vi "ReferencedVariables_AddReferenceVariable.vi"(7 "Action":T2=enum."GeneratePattern", 8 "error in (no error)":errorcluster, 10 "DataIn":variant, 11 "ClassRefToActOn":refnum<vi>) -> (0 "error out":errorcluster, 1 "Name":string, 2 "DataOut":variant, 3 "Cancelled":bool)   [LabVIEW 2014]
uses:
  <resource>/Framework/Providers/Open_GDS/ClassProviders/Provider_BaseClassInterface/BaseProvider_SubVIs/BaseProvider_DesignPatternsActions.ctl
  <resource>/Framework/Providers/Open_GDS/ClassProviders/Common/CommonVIs/CommonVIs_AttributeDataType.ctl
  <resource>/Framework/Providers/Open_GDS/ClassProviders/Common/LvClass_class/GDSLvClass_ProviderTypes.ctl
  <resource>/Framework/Providers/Open_GDS/ClassProviders/Provider_EndevoGOOP300/EndevoProviderName.ctl
  <resource>/Framework/Providers/Open_GDS/ClassProviders/Provider_EndevoGOOP400/EndevoG4ProviderName.ctl
  <resource>/Framework/Providers/Open_GDS/ClassProviders/Provider_LvNativeClass/LvNativeProviderName.ctl
  <resource>/Framework/Providers/Open_GDS/ClassProviders/Common/ScriptingFunctions/Scripting_ConnectorPanePatternType.ctl
  <vilib>/picture/picture.llb/imagedata.ctl
panel:
  in  "_OK+Open":bool
  in  "Delete VI name":string
  in  "Create VI name":string
  out "AlreadyExistsText:VariableName":string
  in  "PlaceInObjectAttribute":bool
  in  "AddViToDelete":bool
  in  "AddViToCreate":bool
  in  "DataType":T1
  in  "Array?":u16(ring) items=["No", "1D", "2D", "3D"]
  in  "Name":string
  in  "_Cancel":bool
  in  "_OK":bool
  out "AlreadyExistsText:Delete":string
  out "AlreadyExistsText:Create":string
  # "Referenced Variables"
  # "Create the variable"
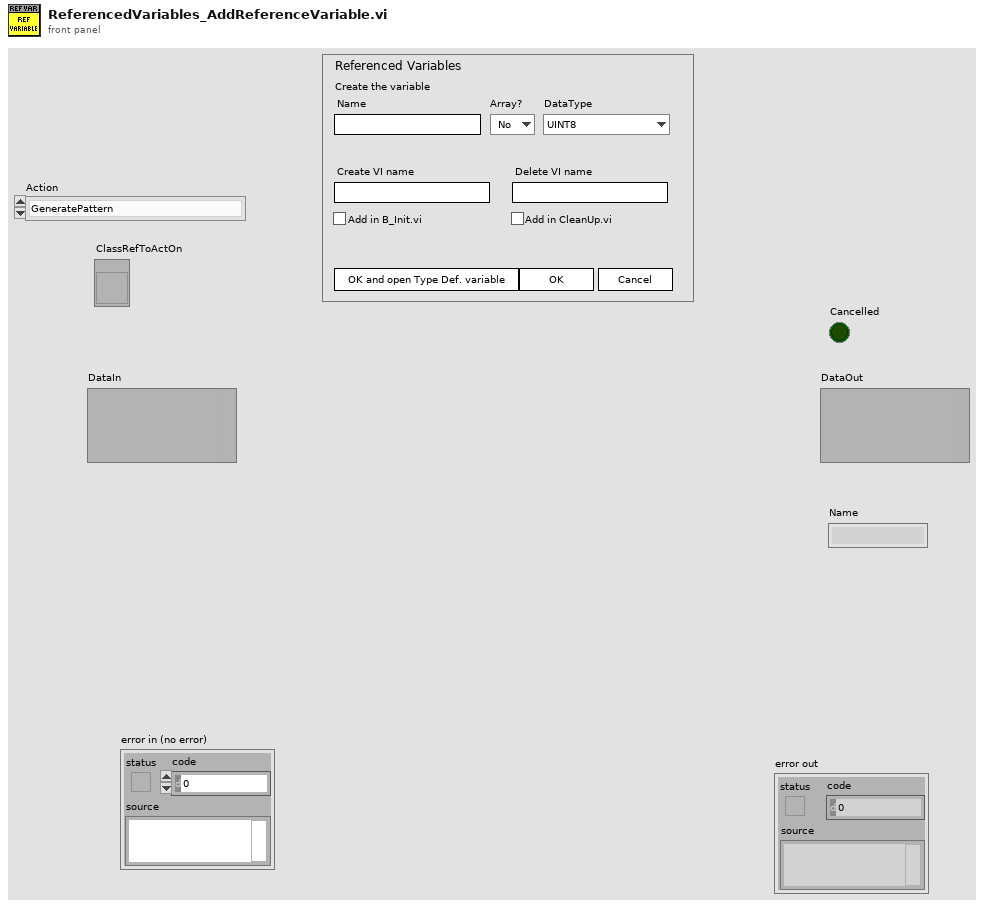
[diagram p1: front panel]
types:
  T1 = typedef "CommonVIs_AttributeDataType.ctl" = enum16{"UINT8", "INT8", "UINT16", "INT16", "UINT32", "INT32", "UINT64", "INT64", "SGL", "DBL", "EXT", "CSG", "CDB", "CXT", "TimeStamp", "STRING", "PATH", "BOOL", "ENUM", "RefNum", "VIRefNum", "LabVIEW Class", "Cluster", "Variant", "TypeDef", "Waveform", "LabVIEW Object", "Other", "void"}
  T2 = typedef "BaseProvider_DesignPatternsActions.ctl" = enum16{"AddPatternDialog", "GeneratePattern", "RemovePattern", "CreatePatternMethod", "UpdatePattern"}
  T3 = cluster{"Name":string, "Array?":u16, "DataType":T1, "Open?":bool, "VarCreateVI":string, "VarDestroyVI":string, "AddViToCreate":bool, "AddViToDelete":bool, "PlaceInObjectAttribute":bool, "ClassCreateVI":string, "ClassDestroyVI":string}
  T4 = typedef "GDSLvClass_ProviderTypes.ctl" = enum16{"UnKnown(LabVOOP)", "Native", "EndevoGOOP3", "OpenG(RootObject)", "OpenG(OpenG_Object)", "EndevoGOOP4", "JKI1"}
  T5 = cluster{"Data":cluster{"Name":string, "Array?":u16, "DataType":T1, "Open?":bool, "VarCreateVI":string, "VarDestroyVI":string, "AddViToCreate":bool, "AddViToDelete":bool, "PlaceInObjectAttribute":bool, "ClassCreateVI":string, "ClassDestroyVI":string}, "SupportFolder":path, "ClassProvider":T4, "ClassName":string, "TemplateName":string, "RefVariablesFolder":path, "Variable.ctl":path, "CreateRefVar.vi":path, "DeleteRefVar.vi":path, "VariablePath":path, "VariableRef":refnum<vi>, "CreateRef":refnum<vi>, "DeleteRef":refnum<vi>, "Application":refnum<vi>, "RefVariablesFolderRef":refnum<vi>, "ClassRef":refnum<vi>, "Singleton":bool, "MethodTemplate":path, "VI":refnum<vi>, "GetObjectStatus":path, "TemplateVI":path, "VI_ToFind":path, "Name":string}
  T6 = enum8{"Enabled", "Disabled", "Disabled and Grayed Out"}
  T7 = typedef "LvNativeProviderName.ctl" = enum16{"Endevo LabVIEW Native"}
  T8 = typedef "EndevoG4ProviderName.ctl" = enum16{"EndevoGOOP400"}
  T9 = typedef "EndevoProviderName.ctl" = enum16{"EndevoGOOP300"}
  T10 = cluster{"Cancelled":bool, "Files":string[], "ClassPath":path, "DataOut":variant, "ByRef":bool, "FilePaths":path[], "CreateVI":string, "DeleteVi":string, "Open?":bool, "Name":string}
  T11 = typedef "imagedata.ctl" = cluster{"image type":i32, "image depth":i32, "image":u8[], "mask":u8[], "colors":u32[], "Rectangle":cluster{"left":i16, "top":i16, "right":i16, "bottom":i16}}
  T12 = typedef "GDSLvCLass_ClassSettingsType.ctl" = cluster{"ClassProviderName":string, "ClassTemplateUsed":string, "ClassTemplateVersion":string, "ClassDescription":string, "PlugIns":T13[], "ConnectorPanePattern":string}
  T13 = typedef "GDSLvClass_PlugIn.ctl" = cluster{"Type":T14, "ID":string, "Version":string, "Path":path, "Name":string, "Data":variant}
  T14 = typedef "GDSLvClass_PlugInTypes.ctl" = enum16{"DesignPattern", "MethodTypes"}
  T15 = typedef "Scripting_ConnectorPanePatternType.ctl" = u16
  T16 = typedef "GDSLvClass_IconSettingsType.ctl" = cluster{"Frame":u32, "Frame thickness":u8, "Header Background":u32, "Header Text":u32, "ColorPublic":u32, "ColorProtected":u32, "ColorPrivate":u32, "Body Text":u32, "ClassBodyIcon":string}
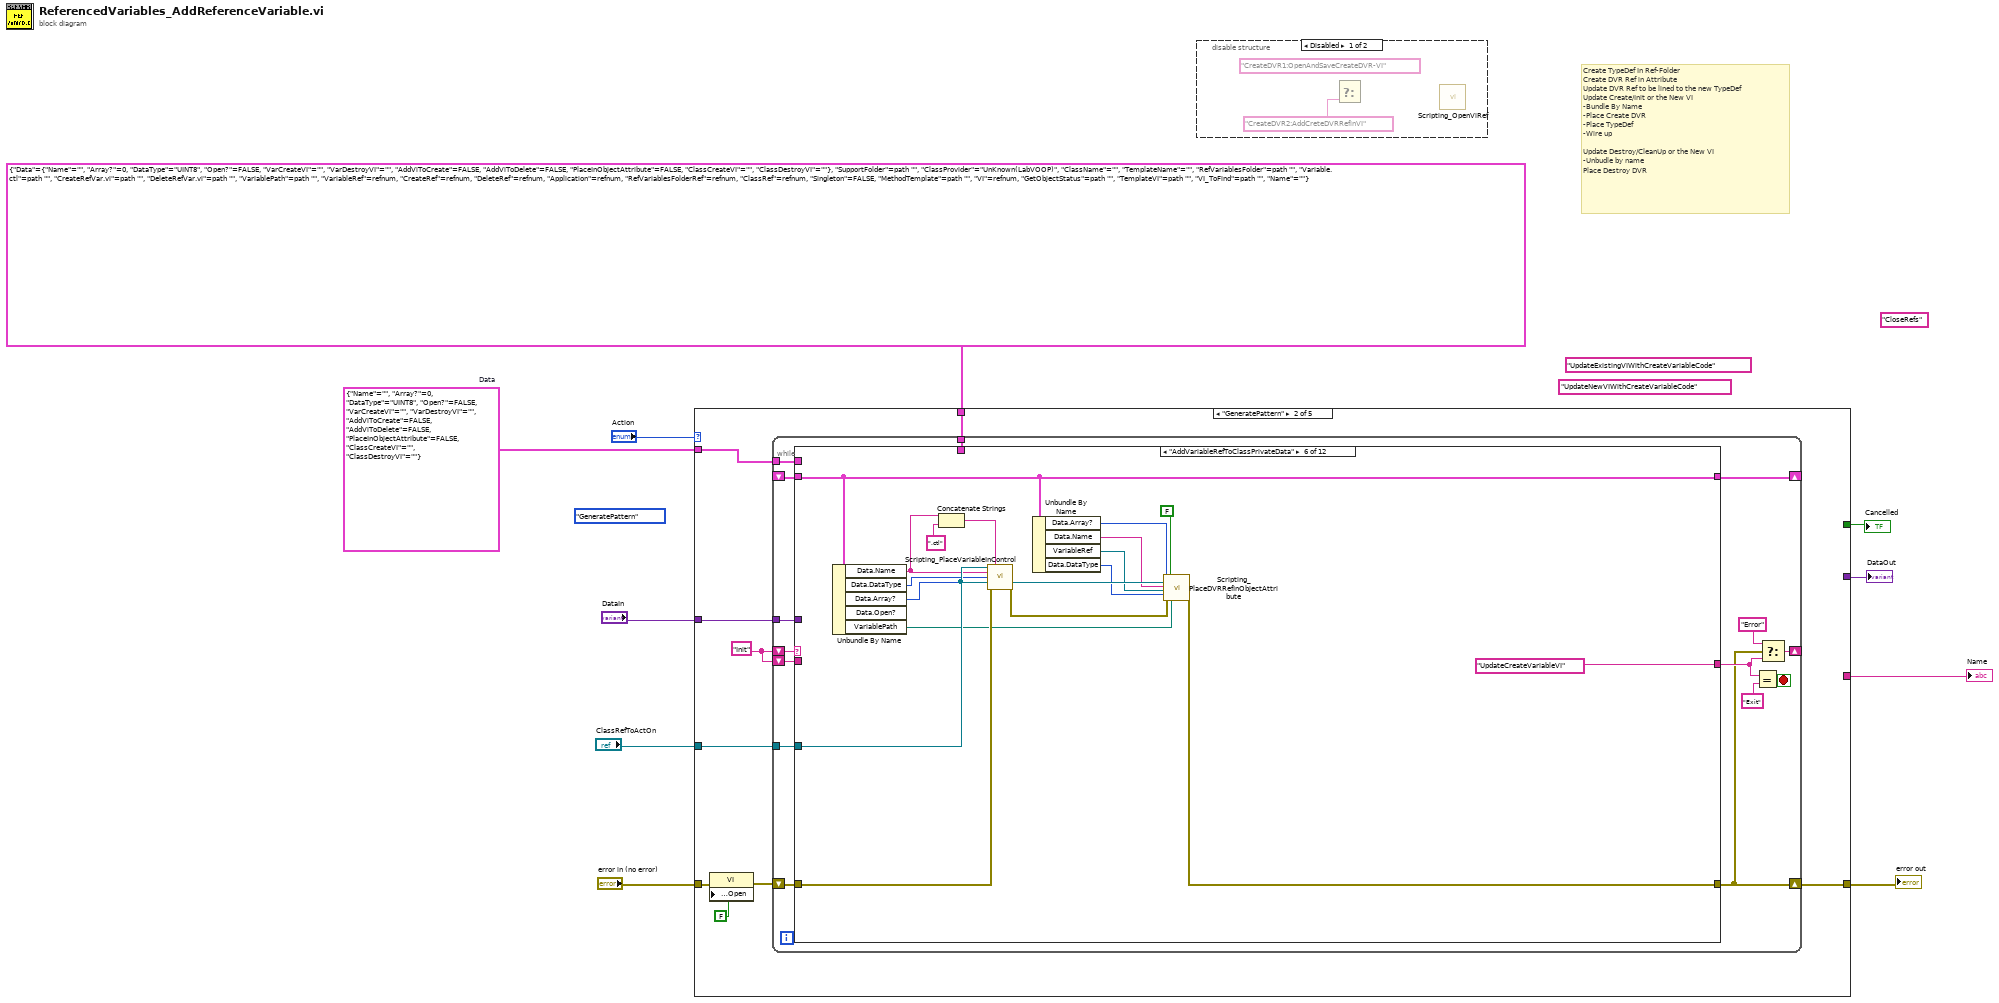
[diagram p0: block diagram]
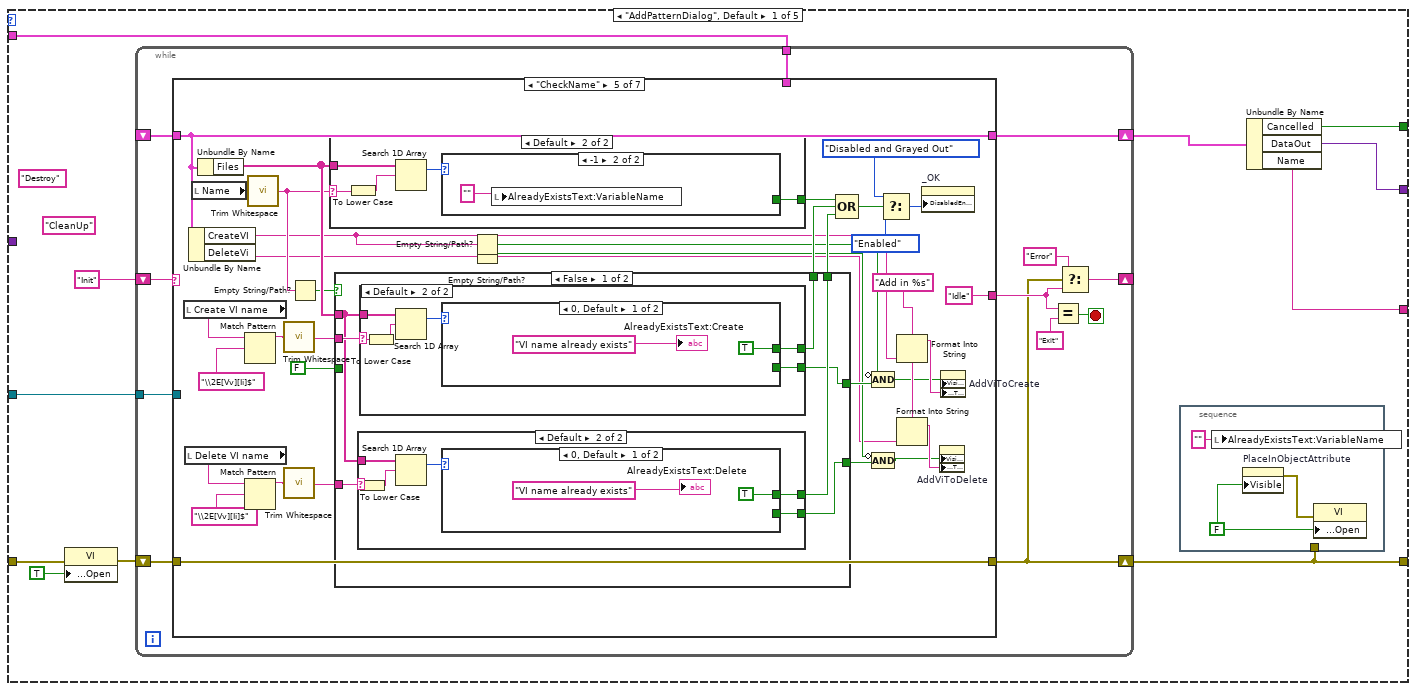
[diagram p3: hidden frame]
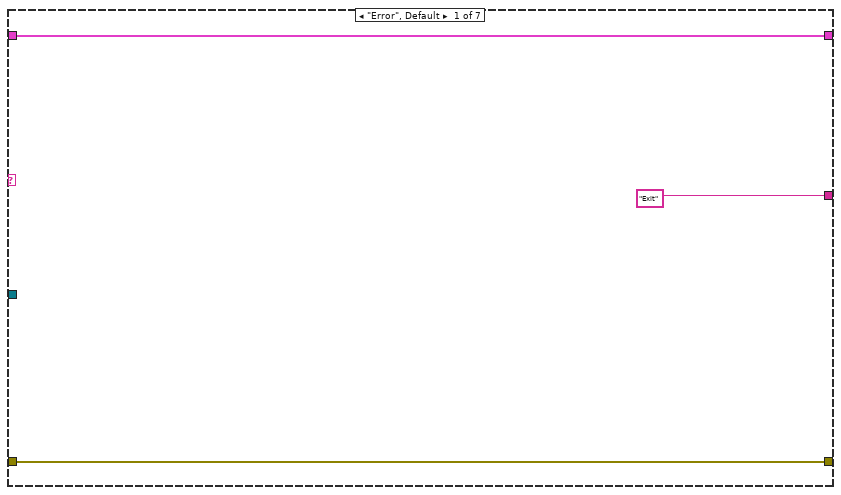
[diagram p4: hidden frame]
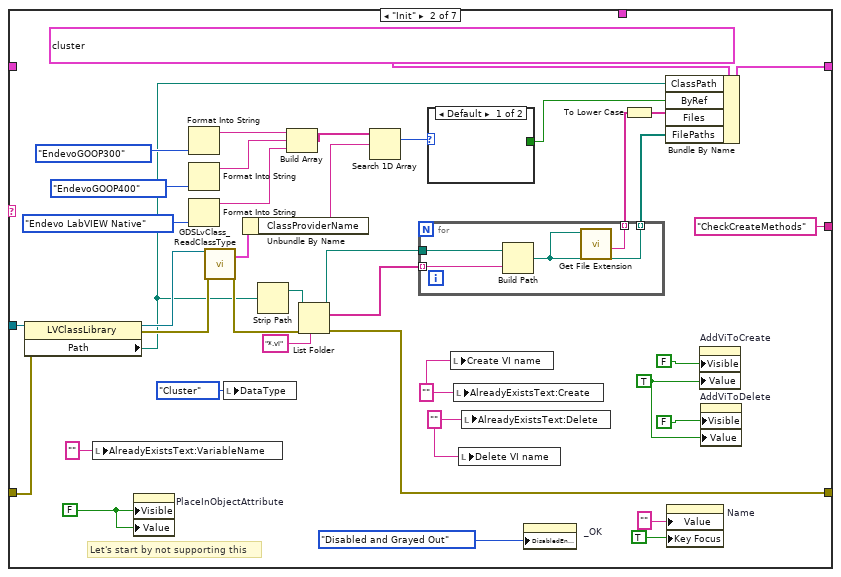
[diagram p5: hidden frame]
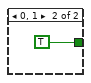
[diagram p6: hidden frame]
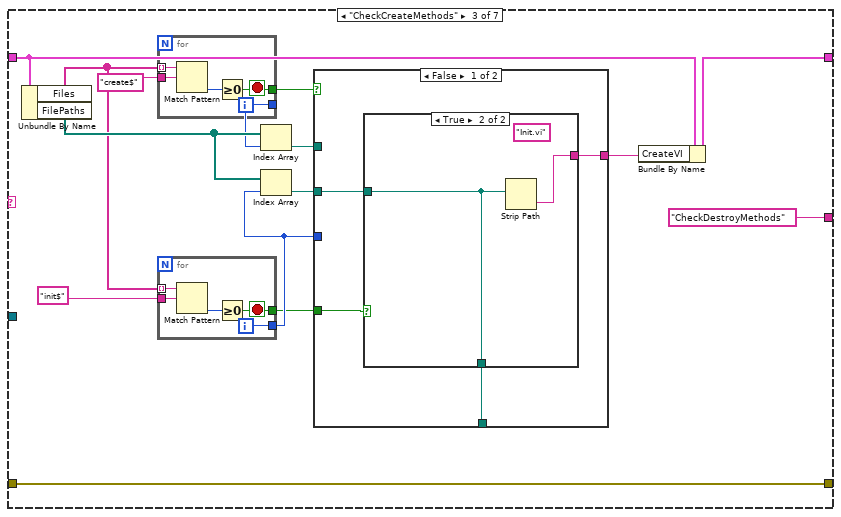
[diagram p7: hidden frame]
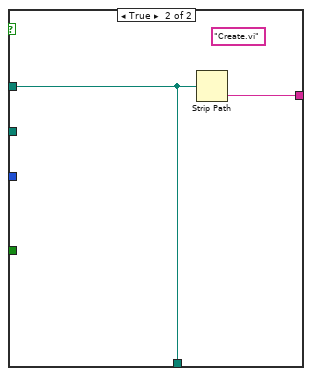
[diagram p9: hidden frame]
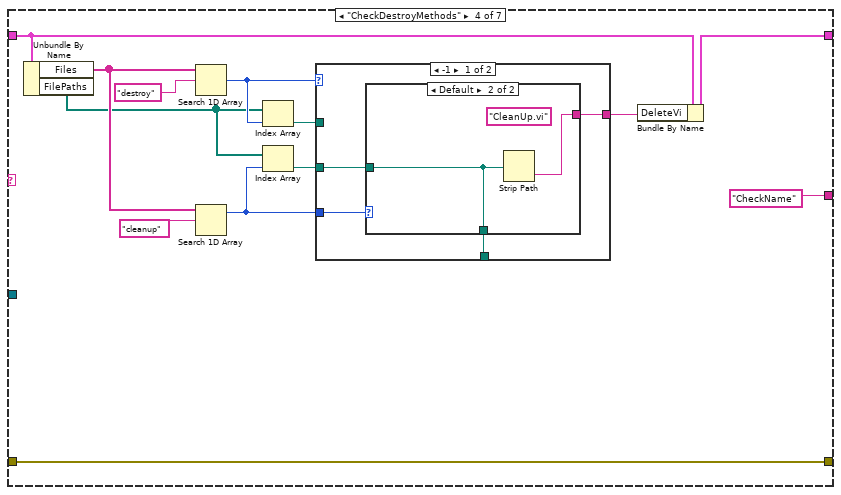
[diagram p10: hidden frame]
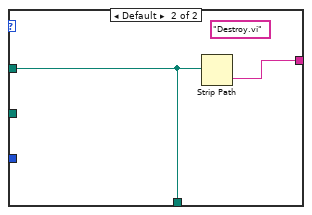
[diagram p12: hidden frame]
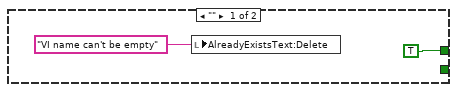
[diagram p13: hidden frame]
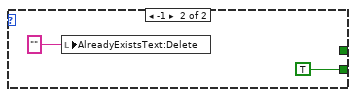
[diagram p14: hidden frame]
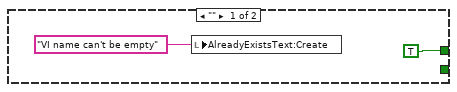
[diagram p15: hidden frame]
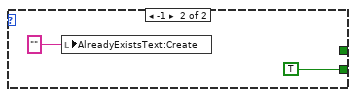
[diagram p16: hidden frame]
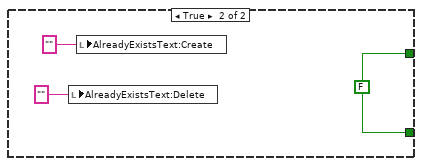
[diagram p17: hidden frame]
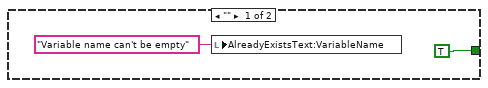
[diagram p18: hidden frame]
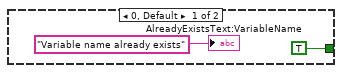
[diagram p19: hidden frame]
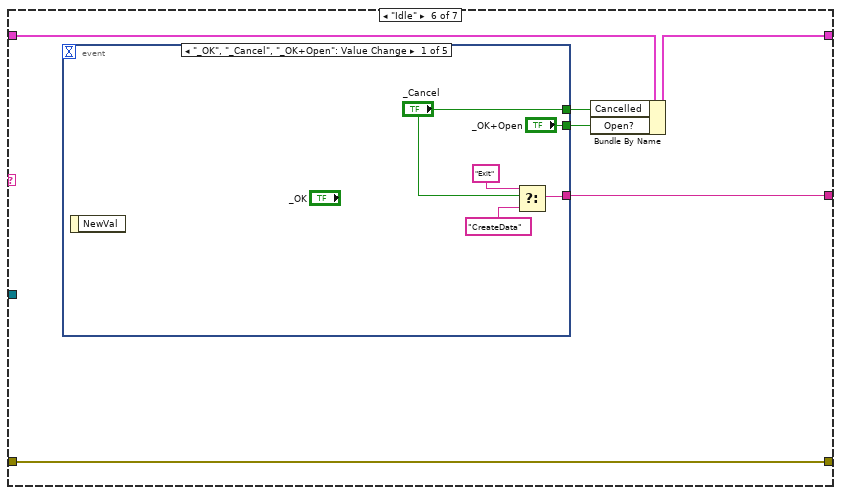
[diagram p20: hidden frame]
diagram:
  (unwired) "CloseRefs"
  (unwired) "UpdateExistingVIWithCreateVariableCode"
  (unwired) "UpdateNewVIWithCreateVariableCode"
  w2 = T3 {"Name"="", "Array?"=0, "DataType"=enum."UINT8", "Open?"=FALSE, "VarCreateVI"="", "VarDestroyVI"="", "AddViToCreate"=FALSE, "AddViToDelete"=FALSE, "PlaceInObjectAttribute"=FALSE, "ClassCreateVI"="", "ClassDestroyVI"=""}  # Data
  (unwired) BaseProvider_DesignPatternsActions."GeneratePattern" ("Action")
  # "Create TypeDef In Ref-Folder\nCreate DVR Ref in Attribute\nUpdate DVR Ref to be lined to the new TypeDef\nUpdate Create/Init or the New VI\n-Bundle By Name\n-Place Create DVR \n-Place TypeDef\n-Wire up\n\nUpdate Destroy/CleanUp or the New VI\n-Unbudle by name\nPlace Destroy DVR"
  n1 = case shown="\"GeneratePattern\"" "Action" {
    tunnel: "error in (no error)" -> [w20 w276 w681 w830 w831]
    tunnel: [w17 w281 w680 w830 w831] -> w9
    tunnel: "ClassRefToActOn" -> [w15 w278 w682 _ _]
    tunnel: [w14 _ _ _ _] -> w7
    tunnel: [w13 _ _ _ _] -> w6
    tunnel: "DataIn" -> [_ w280 w683 _ _]
    tunnel: T5 {"Data"={"Name"="", "Array?"=0, "DataType"=enum."UINT8", "Open?"=FALSE, "VarCreateVI"="", "VarDestroyVI"="", "AddViToCreate"=FALSE, "AddViToDelete"=FALSE, "PlaceInObjectAttribute"=FALSE, "ClassCreateVI"="", "ClassDestroyVI"=""}, "SupportFolder"=path "", "ClassProvider"=enum."UnKnown(LabVOOP)", "ClassName"="", "TemplateName"="", "RefVariablesFolder"=path "", "Variable.ctl"=path "", "CreateRefVar.vi"=path "", "DeleteRefVar.vi"=path "", "VariablePath"=path "", "VariableRef"=refnum, "CreateRef"=refnum, "DeleteRef"=refnum, "Application"=refnum, "RefVariablesFolderRef"=refnum, "ClassRef"=refnum, "Singleton"=FALSE, "MethodTemplate"=path "", "VI"=refnum, "GetObjectStatus"=path "", "TemplateVI"=path "", "VI_ToFind"=path "", "Name"=""} -> [_ w279 w679 _ _]
    tunnel: w2 -> [w12 w273 _ _ _]
    tunnel: [w11 _ _ _ _] -> w1
    frame "AddPatternDialog", Default {
      (unwired) "CleanUp" ("search string")
      (unwired) "Destroy" ("search string")
      n2 = property class="VI"(error in=w20, "Front Panel.Open"=TRUE ("Front Panel Window:Open")) -> (error out=w19:errorcluster)  [unwired: 1 in, 1 out]
      n3 = while {
        shift-right: [w29] -> w17
        shift-left: w19 -> [w36]
        shift-right: [w34] -> _
        shift-left: "Init" -> [w35]
        shift-right: [w28] -> w16
        shift-left: _ -> [w27]
        tunnel: w15 -> [w26]
        tunnel: w12 -> [w25]
        stop <- w33 stop-if-true
        n4 = case shown="\"CheckName\"" w35 {
          tunnel: w36 -> [w39 w74 w90 w118 w171 w220 w270]
          tunnel: [w39 w44 w90 w118 w171 w220 w270] -> w29
          tunnel: ["Exit" "CheckCreateMethods" "CheckDestroyMethods" "CheckName" "Idle" w221 "Exit"] -> w30
          tunnel: [w37 w76 w93 w122 w148 w219 w272] -> w28
          tunnel: w27 -> [w37 _ w94 w123 w148 w217 w245]
          tunnel: w26 -> [_ w75 _ _ _ _ _]
          tunnel: w25 -> [_ _ _ _ _ _ w266]
          frame "Error", Default {
          }
          frame "Init" {
            w50 = "" ("AlreadyExistsText")
            w51 = "" ("AlreadyExistsText")
            w52 = TRUE ("Visible")
            w59 = FALSE ("Visible")
            # "Let's start by not supporting this"
            n5 = property class="LVClassLibrary"(reference=w75, error in=w74) -> (reference out=w72:refnum<vi>, error out=w71:errorcluster, "Path"=w47:path)
            n6 = local write "AlreadyExistsText:VariableName"("" ("AlreadyExistsText")) -> ()
            n7 = property on="PlaceInObjectAttribute" class="Bool (strict)"("Visible"=w59, "Value"=w59) -> ()  [unwired: 2 in, 2 out]
            n8 = Format Into String(EndevoProviderName."EndevoGOOP300" ("ProviderName")) -> (resulting string=w69:string)  [unwired: 3 in, 1 out]
            n9 = Format Into String(EndevoG4ProviderName."EndevoGOOP400" ("ProviderName")) -> (resulting string=w68:string)  [unwired: 3 in, 1 out]
            n10 = Format Into String(LvNativeProviderName."Endevo LabVIEW Native" ("ProviderName")) -> (resulting string=w67:string)  [unwired: 3 in, 1 out]
            n11 = call <resource>:"GDSLvClass_ReadClassType.vi"("Class Refnum In"=w72, "error in (no error)"=w71) -> ("ClassSettings"=w73:T12, "error out"=w49:errorcluster)  [unwired: 15 in, 1 out]
            n12 = local write "DataType"(CommonVIs_AttributeDataType."Cluster" ("DataType")) -> ()
            n13 = Unbundle By Name(w73) -> ("ClassProviderName"=w65:string)
            n14 = Strip Path(path=w47) -> (stripped path=w46:path)  [unwired: 1 out]
            n15 = Build Array(w69, w68, w67) -> (w66:string[])
            n16 = List Folder(path=w46, pattern="*.vi", error in=w49) -> (path out=w45:path, filenames=w42:string[], error out=w44:errorcluster)  [unwired: 1 in, 1 out]
            n17 = Search 1D Array(1D array=w66, element=w65) -> (index of element=w64:i32)  [unwired: 1 in]
            n18 = for {
              tunnel: [w81] -> w58 mode=indexing
              tunnel: w45 -> [w83]
              tunnel: w42 -> [w82] mode=indexing
              tunnel: [w80] -> w41 mode=indexing
              n19 = Build Path(base path=w83, name or relative path=w82) -> (appended path=w81:path)
              n20 = call <vilib>:"Get File Extension.vi"("file"=w81) -> ("filename without extension"=w80:string)  [unwired: 7 in, 3 out]
            }
            n21 = case shown="Default" w64 {
              tunnel: [_ TRUE] -> w61
              frame Default {
              }
              frame 0, 1 {
              }
            }
            n22 = local write "Create VI name"(w51) -> ()
            n23 = local write "AlreadyExistsText:Create"(w51) -> ()
            n24 = local write "Delete VI name"(w50) -> ()
            n25 = local write "AlreadyExistsText:Delete"(w50) -> ()
            n26 = property on="_OK" class="Bool"("DisabledEnum"=T6."Disabled and Grayed Out" ("Disabled")) -> ()  [unwired: 2 in, 2 out]
            n27 = To Lower Case(string=w41) -> (all lower case string=w43:string[])
            n28 = Bundle By Name(cluster=T10 {"Cancelled"=FALSE, "Files"=[], "ClassPath"=path "", "DataOut"=variant, "ByRef"=FALSE, "FilePaths"=[], "CreateVI"="", "DeleteVi"="", "Open?"=TRUE, "Name"=""}, "ClassPath"=w47, "ByRef"=w61, "Files"=w43, "FilePaths"=w58) -> (w76:T10)
            n29 = property on="Name" class="Str"("Value"="" ("AlreadyExistsText"), "Key Focus"=TRUE) -> ()  [unwired: 2 in, 2 out]
            n30 = property on="AddViToCreate" class="Bool (strict)"("Visible"=FALSE, "Value"=w52) -> ()  [unwired: 2 in, 2 out]
            n31 = property on="AddViToDelete" class="Bool (strict)"("Visible"=FALSE, "Value"=w52) -> ()  [unwired: 2 in, 2 out]
          }
          frame "CheckCreateMethods" {
            n32 = Unbundle By Name(w94) -> ("Files"=w87:string[], "FilePaths"=w96:path[])
            n33 = for {
              tunnel: w87 -> [w108] mode=indexing
              tunnel: "create$" ("search string") -> [w107]
              tunnel: [w105] -> w91
              tunnel: [w104] -> w88
              i -> [w105]
              stop <- w104 stop-if-true
              n34 = Match Pattern(string=w108, regular expression=w107) -> (offset past match=w106:i32)  [unwired: 1 in, 3 out]
              n35 = Greater Or Equal To 0?(x=w106) -> (x >= 0?=w104:bool)
            }
            n36 = for {
              tunnel: w87 -> [w103] mode=indexing
              tunnel: "init$" ("search string") -> [w102]
              tunnel: [w100] -> w85
              tunnel: [w99] -> w84
              i -> [w100]
              stop <- w99 stop-if-true
              n37 = Match Pattern(string=w103, regular expression=w102) -> (offset past match=w101:i32)  [unwired: 1 in, 3 out]
              n38 = Greater Or Equal To 0?(x=w101) -> (x >= 0?=w99:bool)
            }
            n39 = Index Array(array=w96, index=w91) -> (element=w97:path)
            n40 = Index Array(array=w96, index=w85) -> (element=w95:path)
            n41 = case shown="False" w88 {
              tunnel: w85 -> [_ _]
              tunnel: [w111 w116] -> _
              tunnel: w97 -> [_ w116]
              tunnel: w95 -> [w112 _]
              tunnel: [w110 w115] -> w89
              tunnel: w84 -> [w109 _]
              frame False {
                n42 = case shown="True" w109 {
                  tunnel: w112 -> [_ w114]
                  tunnel: [_ w114] -> w111
                  tunnel: [_ w113] -> w110
                  frame False {
                  }
                  frame True {
                    (unwired) "Init.vi" ("search string")
                    n43 = Strip Path(path=w114) -> (name=w113:string)  [unwired: 1 out]
                  }
                }
              }
              frame True {
                (unwired) "Create.vi" ("search string")
                n44 = Strip Path(path=w116) -> (name=w115:string)  [unwired: 1 out]
              }
            }
            n45 = Bundle By Name(cluster=w94, "CreateVI"=w89) -> (w93:T10)
          }
          frame "CheckDestroyMethods" {
            n46 = Unbundle By Name(w123) -> ("Files"=w128:string[], "FilePaths"=w120:path[])
            n47 = Search 1D Array(1D array=w128, element="destroy" ("search string")) -> (index of element=w125:i32)  [unwired: 1 in]
            n48 = Search 1D Array(1D array=w128, element="cleanup" ("search string")) -> (index of element=w121:i32)  [unwired: 1 in]
            n49 = Index Array(array=w120, index=w125) -> (element=w124:path)
            n50 = Index Array(array=w120, index=w121) -> (element=w119:path)
            n51 = case shown="-1" w125 {
              tunnel: w121 -> [w133 _]
              tunnel: [w131 w137] -> _
              tunnel: w124 -> [_ w137]
              tunnel: w119 -> [w132 _]
              tunnel: [w130 w136] -> w117
              frame -1 {
                n52 = case shown="Default" w133 {
                  tunnel: w132 -> [_ w135]
                  tunnel: [_ w135] -> w131
                  tunnel: [_ w134] -> w130
                  frame -1 {
                  }
                  frame Default {
                    (unwired) "CleanUp.vi" ("search string")
                    n53 = Strip Path(path=w135) -> (name=w134:string)  [unwired: 1 out]
                  }
                }
              }
              frame Default {
                (unwired) "Destroy.vi" ("search string")
                n54 = Strip Path(path=w137) -> (name=w136:string)  [unwired: 1 out]
              }
            }
            n55 = Bundle By Name(cluster=w123, "DeleteVi"=w117) -> (w122:T10)
          }
          frame "CheckName" {
            w151 = "Add in %s" ("format string")
            n56 = local read "Create VI name"() -> (w141:string)
            n57 = local read "Delete VI name"() -> (w138:string)
            n58 = Unbundle By Name(w148) -> ("CreateVI"=w140:string, "DeleteVi"=w139:string)
            n59 = local read "Name"() -> (w162:string)
            n60 = Unbundle By Name(w148) -> ("Files"=w155:string[])
            n61 = Match Pattern(string=w141, regular expression="\\2E[Vv][Ii]$") -> (before substring=w163:string)  [unwired: 1 in, 3 out]
            n62 = Match Pattern(string=w138, regular expression="\\2E[Vv][Ii]$") -> (before substring=w159:string)  [unwired: 1 in, 3 out]
            n63 = call <vilib>:"Trim Whitespace.vi"("string"=w162) -> ("trimmed string"=w154:string)  [unwired: 1 in]
            n64 = call <vilib>:"Trim Whitespace.vi"("string"=w163) -> ("trimmed string"=w161:string)  [unwired: 1 in]
            n65 = call <vilib>:"Trim Whitespace.vi"("string"=w159) -> ("trimmed string"=w160:string)  [unwired: 1 in]
            n66 = Empty String/Path?(string/path=w154) -> (empty?=w153:bool)
            n67 = case shown="Default" w154 {
              selector: w154 -> [_ w208]
              tunnel: w155 -> [_ w210]
              tunnel: [TRUE w209] -> w168
              frame "" {
                n68 = local write "AlreadyExistsText:VariableName"("Variable name can't be empty" ("AlreadyExistsText")) -> ()
              }
              frame Default {
                n69 = To Lower Case(string=w208) -> (all lower case string=w211:string)
                n70 = Search 1D Array(1D array=w210, element=w211) -> (index of element=w212:i32)  [unwired: 1 in]
                n71 = case shown="-1" w212 {
                  tunnel: [TRUE _] -> w209
                  frame 0, Default {
                    "AlreadyExistsText:VariableName" <- "Variable name already exists" ("AlreadyExistsText")
                  }
                  frame -1 {
                    n72 = local write "AlreadyExistsText:VariableName"("" ("AlreadyExistsText")) -> ()
                  }
                }
              }
            }
            n73 = case shown="False" w153 {
              tunnel: w161 -> [w178 _]
              tunnel: w160 -> [w177 _]
              tunnel: [w176 _] -> w157
              tunnel: [w175 _] -> w156
              tunnel: w155 -> [w174 _]
              tunnel: FALSE ("x = 0?") -> [_ _]
              tunnel: [w173 w203] -> w147
              tunnel: [w172 w203] -> w144
              frame False {
                n74 = case shown="Default" w177 {
                  selector: w177 -> [_ w182]
                  tunnel: w174 -> [_ w184]
                  tunnel: [TRUE w183] -> w175
                  tunnel: [_ w181] -> w172
                  frame "" {
                    n75 = local write "AlreadyExistsText:Delete"("VI name can't be empty" ("AlreadyExistsText")) -> ()
                  }
                  frame Default {
                    n76 = To Lower Case(string=w182) -> (all lower case string=w185:string)
                    n77 = Search 1D Array(1D array=w184, element=w185) -> (index of element=w186:i32)  [unwired: 1 in]
                    n78 = case shown="0, Default" w186 {
                      tunnel: [TRUE _] -> w183
                      tunnel: [_ TRUE] -> w181
                      frame 0, Default {
                        "AlreadyExistsText:Delete" <- "VI name already exists" ("AlreadyExistsText")
                      }
                      frame -1 {
                        n79 = local write "AlreadyExistsText:Delete"("" ("AlreadyExistsText")) -> ()
                      }
                    }
                  }
                }
                n80 = case shown="Default" w178 {
                  selector: w178 -> [_ w194]
                  tunnel: w174 -> [_ w196]
                  tunnel: [TRUE w195] -> w176
                  tunnel: [_ w193] -> w173
                  frame "" {
                    n81 = local write "AlreadyExistsText:Create"("VI name can't be empty" ("AlreadyExistsText")) -> ()
                  }
                  frame Default {
                    n82 = To Lower Case(string=w194) -> (all lower case string=w197:string)
                    n83 = Search 1D Array(1D array=w196, element=w197) -> (index of element=w198:i32)  [unwired: 1 in]
                    n84 = case shown="0, Default" w198 {
                      tunnel: [TRUE _] -> w195
                      tunnel: [_ TRUE] -> w193
                      frame 0, Default {
                        "AlreadyExistsText:Create" <- "VI name already exists" ("AlreadyExistsText")
                      }
                      frame -1 {
                        n85 = local write "AlreadyExistsText:Create"("" ("AlreadyExistsText")) -> ()
                      }
                    }
                  }
                }
              }
              frame True {
                w203 = FALSE
                n86 = local write "AlreadyExistsText:Delete"("" ("AlreadyExistsText")) -> ()
                n87 = local write "AlreadyExistsText:Create"("" ("AlreadyExistsText")) -> ()
              }
            }
            n88 = Empty String/Path?(string/path=w140) -> (empty?=w145:bool)
            n89 = Empty String/Path?(string/path=w139) -> (empty?=w142:bool)
            n90 = Compound Arithmetic op=OR(w168, w157, w156) -> (w167:bool)
            n91 = Compound Arithmetic op=AND(invert w145, w147) -> (w146:bool)
            n92 = Compound Arithmetic op=AND(invert w142, w144) -> (w143:bool)
            n93 = Select(t=T6."Disabled and Grayed Out" ("Disabled"), s=w167, f=T6."Enabled" ("Disabled")) -> (s? t:f=w164:T6)
            n94 = Format Into String(format string=w151, w140) -> (resulting string=w150:string)  [unwired: 2 in, 1 out]
            n95 = Format Into String(format string=w151, w139) -> (resulting string=w149:string)  [unwired: 2 in, 1 out]
            n96 = property on="_OK" class="Bool"("DisabledEnum"=w164) -> ()  [unwired: 2 in, 2 out]
            n97 = property on="AddViToDelete" class="Bool (strict)"("Visible"=w143, "BoolText.Text"=w149) -> ()  [unwired: 2 in, 2 out]
            n98 = property on="AddViToCreate" class="Bool (strict)"("Visible"=w146, "BoolText.Text"=w150) -> ()  [unwired: 2 in, 2 out]
          }
          frame "Idle" {
            n99 = event shown="[0] \"_OK\", \"_Cancel\", \"_OK+Open\": Value Change" {
              selector: _ -> [_ _ _ _ _]
              dyn-events: _ -> [_ _ _ _ _]
              timeout: _ -> [_ _ _ _ _]
              tunnel: [w226 "Exit" "CheckName" "CheckName" "CheckName"] -> w221
              tunnel: ["_Cancel" w227 _ _ _] -> w218
              tunnel: ["_OK+Open" _ _ _ _] -> w216
              event "_OK", "_Cancel", "_OK+Open": Value Change {
                n100 = event-data() -> ()  [unwired: 1 in, 1 out]
                n101 = Select(t="Exit", s="_Cancel", f="CreateData") -> (s? t:f=w226:string)
              }
              event Panel Close? {
                w227 = TRUE ("Discard?")
                n102 = event-data() -> ()  [unwired: 1 in, 1 out]
                n103 = event-data("Discard?"=w227) -> ()  [unwired: 1 in, 1 out]
              }
              event "Name": Value Change {
                n104 = event-data() -> ()  [unwired: 1 in, 1 out]
                n105 = Empty String/Path?(string/path="Name") -> (empty?=w229:bool)
                n106 = case shown="False" w229 {
                  tunnel: [w239 _] -> w232
                  tunnel: [w238 _] -> w231
                  tunnel: "Name" -> [w236 _]
                  frame False {
                    n107 = Concatenate Strings("Create" ("string"), w236, "Ref" ("string")) -> (w239:string)
                    n108 = Concatenate Strings("Delete" ("string"), w236, "Ref" ("string")) -> (w238:string)
                  }
                  frame True {
                  }
                }
                n109 = local write "Delete VI name"(w231) -> ()
                n110 = local write "Create VI name"(w232) -> ()
              }
              event "Create VI name", "Delete VI name": Value Change {
                n111 = event-data() -> ()  [unwired: 1 in, 1 out]
              }
              event "AddViToDelete", "AddViToCreate": Value Change {
                n112 = event-data() -> ()  [unwired: 1 in, 1 out]
              }
            }
            n113 = Bundle By Name(cluster=w217, "Cancelled"=w218, "Open?"=w216) -> (w219:T10)
          }
          frame "CreateData" {
            # "Hidden for now"
            n114 = Unbundle By Name(w245) -> ("Open?"=w244:bool)
            n115 = local read "Create VI name"() -> (w263:string)
            n116 = local read "Delete VI name"() -> (w257:string)
            n117 = local read "AddViToDelete"() -> (w250:bool)
            n118 = Unbundle By Name(w245) -> ("CreateVI"=w247:string, "DeleteVi"=w246:string)
            n119 = local read "AddViToCreate"() -> (w251:bool)
            n120 = local read "Name"() -> (w265:string)
            n121 = call <vilib>:"Trim Whitespace.vi"("string"=w263) -> ("trimmed string"=w262:string)  [unwired: 1 in]
            n122 = call <vilib>:"Trim Whitespace.vi"("string"=w257) -> ("trimmed string"=w256:string)  [unwired: 1 in]
            n123 = Match Pattern(string=w262, regular expression="\\2E[Vv][Ii]$") -> (before substring=w261:string)  [unwired: 1 in, 3 out]
            n124 = Match Pattern(string=w256, regular expression="\\2E[Vv][Ii]$") -> (before substring=w255:string)  [unwired: 1 in, 3 out]
            n125 = call <vilib>:"Trim Whitespace.vi"("string"=w265) -> ("trimmed string"=w243:string)  [unwired: 1 in]
            n126 = call <vilib>:"Trim Whitespace.vi"("string"=w261) -> ("trimmed string"=w260:string)  [unwired: 1 in]
            n127 = call <vilib>:"Trim Whitespace.vi"("string"=w255) -> ("trimmed string"=w254:string)  [unwired: 1 in]
            n128 = Concatenate Strings(w260, ".vi" ("string")) -> (w248:string)
            n129 = Concatenate Strings(w254, ".vi" ("string")) -> (w252:string)
            n130 = Bundle(cluster=w266, "Name"=w243, "Array?"="Array?", "DataType"="DataType", "Open?"=w244, "VarCreateVI"=w248, "VarDestroyVI"=w252, "AddViToCreate"=w251, "AddViToDelete"=w250, "PlaceInObjectAttribute"="PlaceInObjectAttribute", "ClassCreateVI"=w247, "ClassDestroyVI"=w246) -> (w267:T3)
            n131 = Bundle By Name(cluster=w245, "Name"=w243, "DataOut"=w267) -> (w272:T10)
          }
        }
        n132 = Equal?(x=w30, y="Exit") -> (x = y?=w33:bool)
        n133 = Select(t="Error", s=w29, f=w30) -> (s? t:f=w34:string)
      }
      n134 = stacked-sequence {
        tunnel: w17 -> [_]
        frame #0 {
          w24 = FALSE ("Front Panel Window:Open")
          n135 = local write "AlreadyExistsText:VariableName"("" ("AlreadyExistsText")) -> ()
          n136 = property on="PlaceInObjectAttribute" class="Bool (strict)"("Visible"=w24) -> (error out=w23:errorcluster)  [unwired: 2 in, 1 out]
          n137 = property class="VI"(error in=w23, "Front Panel.Open"=w24) -> ()  [unwired: 1 in, 2 out]
        }
      }
      n138 = Unbundle By Name(w16) -> ("Cancelled"=w14:bool, "DataOut"=w13:variant, "Name"=w11:string)
    }
    frame "GeneratePattern" {
      w274 = "Init"
      n139 = property class="VI"(error in=w276, "Front Panel.Open"=FALSE ("Front Panel Window:Open")) -> (error out=w275:errorcluster)  [unwired: 1 in, 1 out]
      n140 = while {
        shift-right: [w289] -> w281
        shift-left: w275 -> [w296]
        shift-right: [w294] -> _
        shift-left: w274 -> [w295]
        shift-right: [w288] -> _
        shift-left: _ -> [w287]
        tunnel: w280 -> [w286]
        tunnel: w273 -> [w285]
        tunnel: w279 -> [w284]
        tunnel: w278 -> [w283]
        shift-left: w274 -> [w282]
        stop <- w293 stop-if-true
        n141 = case shown="\"AddVariableRefToClassPrivateData\"" w295 {
          tunnel: w296 -> [w321 w363 w379 w395 w412 w430 w456 w486 w500 w541 w595 w661]
          tunnel: [w302 w358 w375 w389 w404 w429 w436 w467 w499 w540 w594 w665] -> w289
          tunnel: ["GetTemplateVIs" "OpenTemplateVIs" "SaveVIToNewName" "AddVIsToClass" "AddVariableRefToClassPrivateData" "UpdateCreateVariableVI" "UpdateDeleteVariableVI" "UpdateIcons" "AddCreateVariableVIInCreate" "AddDeleteVariableVIInDestroy" "CloseRefs" "Exit"] -> w290
          tunnel: [w325 w348 w370 w386 w402 w414 w443 w474 w501 w536 w590 w663] -> w288
          tunnel: w287 -> [_ w362 w369 w387 w402 w414 w443 w474 w501 w536 w590 w663]
          tunnel: w286 -> [w324 _ _ _ _ _ _ _ _ _ _ _]
          tunnel: w285 -> [w323 _ _ _ _ _ _ _ _ _ _ _]
          tunnel: w284 -> [w322 _ _ _ _ _ _ _ _ _ _ _]
          tunnel: w283 -> [w320 w364 _ _ _ w428 _ _ w503 w537 w591 w659]
          tunnel: w282 -> [_ _ _ _ _ _ _ _ _ _ _ w662]
          frame "Init" {
            w300 = "ReferencedVariables" ("name or relative path")
            n142 = Variant To Data(error in=w321, type=w323, Variant=w324) -> (data=w306:T3, error out=w315:errorcluster)
            n143 = property class="LVClassLibrary"(reference=w320, error in=w315) -> (reference out=w297:refnum<vi>, error out=w307:errorcluster, "Path"=w314:path)
            n144 = property class="LVClassLibrary"(reference=w297, error in=w307) -> (reference out=w311:refnum<vi>, error out=w309:errorcluster, "Target"=w310:refnum<vi>)
            n145 = Current VI's Path() -> (path=w318:path)
            n146 = Strip Path(path=w318) -> (stripped path=w317:path)  [unwired: 1 out]
            n147 = To More Generic Class(target class=refnum<vi> refnum ("AddItem"), reference=w297) -> (generic class reference=w301:refnum<vi>)
            n148 = Strip Path(path=w314) -> (stripped path=w305:path, name=w312:string)
            n149 = Build Path(base path=w317, name or relative path="ReferencedVariables_SubVIs") -> (appended path=w313:path)
            n150 = case shown="Error" w309 {
              selector: w309 -> [w328 _]
              tunnel: w310 -> [w332 _]
              tunnel: [w331 w334] -> w308
              tunnel: [w327 w335] -> w303
              tunnel: w311 -> [_ w340]
              tunnel: w307 -> [_ w339]
              frame No Error {
                n151 = property class="TargetItem"(reference=w332, error in=w328) -> (reference out=w329:refnum<vi>, error out=w330:errorcluster, "Context"=w331:refnum<vi>)
                n152 = Close Reference(reference=w329, error in (no error)=w330) -> (error out=w327:errorcluster)
              }
              frame Error {
                n153 = property class="LVClassLibrary"(reference=w340, error in=w339) -> (error out=w333:errorcluster, "Project"=w338:refnum<vi>)  [unwired: 1 out]
                n154 = property class="Project"(reference=w338, error in=w333) -> (reference out=w336:refnum<vi>, error out=w337:errorcluster, "App Ref"=w334:refnum<vi>)
                n155 = Close Reference(reference=w336, error in (no error)=w337) -> (error out=w335:errorcluster)
              }
            }
            n156 = Build Path(base path=w305, name or relative path=w300) -> (appended path=w304:path)
            n157 = call <resource>:"GDSProject_CreateFolder.vi"("Project Item To Create Folder Below(Use MyComputer if not wired)"=w301, "FolderName"=w300, "error in (no error)"=w303, "CreateThePhysicalFolderIfPossible(False)"=TRUE) -> ("ItemOut"=w299:refnum<vi>, "error out"=w302:errorcluster)  [unwired: 12 in, 2 out]
            n158 = Bundle By Name(cluster=w322, "Data"=w306, "SupportFolder"=w313, "ClassName"=w312, "RefVariablesFolder"=w304, "RefVariablesFolderRef"=w299, "Application"=w308, "ClassRef"=w297) -> (w325:T5)
          }
          frame "GetTemplateVIs" {
            w354 = T15 0 items=["4x4x4", "5x6x5", "6x8x6"] ("Pattern")
            n159 = call <resource>:"GDSLvClass_GetClassProviderInformation.vi"("Class Refnum In"=w364, "error in (no error)"=w363) -> ("Class Refnum Out"=w360:refnum<vi>, "ClassProvider"=w361:T4, "error out"=w359:errorcluster)  [unwired: 15 in]
            n160 = Unbundle By Name(w362) -> ("SupportFolder"=w344:path)
            n161 = call <resource>:"GDSLvClass_ReadClassType.vi"("Class Refnum In"=w360, "error in (no error)"=w359) -> ("ClassSettings"=w357:T12, "error out"=w358:errorcluster)  [unwired: 15 in, 1 out]
            n162 = Unbundle By Name(w357) -> ("ConnectorPanePattern"=w350:string, "ClassTemplateUsed"=w356:string)
            n163 = Scan From String(input string=w350, default 1=w354) -> (output 1=w351:T15)  [unwired: 3 in, 3 out]
            n164 = case shown="Default" w351 {
              tunnel: ["4x4x4" "6x8x6"] -> w346
              frame 0 {
              }
              frame Default {
              }
            }
            n165 = Format Into String(format string="ReferencedVariables_CreateReferenceVariable_%s.vi" ("name or relative path"), w346) -> (resulting string=w352:string)  [unwired: 2 in, 1 out]
            n166 = Format Into String(format string="ReferencedVariables_DeleteReferenceVariable_%s.vi" ("name or relative path"), w346) -> (resulting string=w343:string)  [unwired: 2 in, 1 out]
            n167 = Build Path(base path=w344, name or relative path="ReferencedVariable.ctl") -> (appended path=w355:path)
            n168 = Build Path(base path=w344, name or relative path=w352) -> (appended path=w345:path)
            n169 = Build Path(base path=w344, name or relative path=w343) -> (appended path=w342:path)
            n170 = Bundle By Name(cluster=w362, "Variable.ctl"=w355, "ClassProvider"=w361, "CreateRefVar.vi"=w345, "DeleteRefVar.vi"=w342, "TemplateName"=w356) -> (w348:T5)
          }
          frame "OpenTemplateVIs" {
            n171 = Unbundle By Name(w369) -> ("Application"=w376:refnum<vi>, "Variable.ctl"=w380:path)
            n172 = Unbundle By Name(w369) -> ("CreateRefVar.vi"=w368:path)
            n173 = Unbundle By Name(w369) -> ("DeleteRefVar.vi"=w367:path)
            n174 = Open VI Reference(application reference (local)=w376, vi path=w380, error in (no error)=w379) -> (vi reference=w373:refnum<vi>, error out=w378:errorcluster)  [unwired: 3 in]
            n175 = Open VI Reference(application reference (local)=w376, vi path=w368, error in (no error)=w378) -> (vi reference=w372:refnum<vi>, error out=w377:errorcluster)  [unwired: 3 in]
            n176 = Open VI Reference(application reference (local)=w376, vi path=w367, error in (no error)=w377) -> (vi reference=w371:refnum<vi>, error out=w375:errorcluster)  [unwired: 3 in]
            n177 = Bundle By Name(cluster=w369, "VariableRef"=w373, "CreateRef"=w372, "DeleteRef"=w371) -> (w370:T5)
          }
          frame "SaveVIToNewName" {
            n178 = Unbundle By Name(w387) -> ("VariableRef"=w399:refnum<vi>, "RefVariablesFolder"=w384:path, "Data.Name"=w398:string)
            n179 = Unbundle By Name(w387) -> ("CreateRef"=w393:refnum<vi>, "Data.VarCreateVI"=w385:string)
            n180 = Unbundle By Name(w387) -> ("DeleteRef"=w392:refnum<vi>, "Data.VarDestroyVI"=w383:string)
            n181 = Concatenate Strings(w398, ".ctl" ("string")) -> (w396:string)
            n182 = Build Path(base path=w384, name or relative path=w396) -> (appended path=w388:path)
            n183 = Build Path(base path=w384, name or relative path=w385) -> (appended path=w382:path)
            n184 = Build Path(base path=w384, name or relative path=w383) -> (appended path=w381:path)
            n185 = invoke class="VI" method="Save.Instrument"(reference=w399, error in=w395, "Path to saved file"=w388) -> (error out=w394:errorcluster)  [unwired: 3 in, 5 out]
            n186 = invoke class="VI" method="Save.Instrument"(reference=w393, error in=w394, "Path to saved file"=w382) -> (error out=w391:errorcluster)  [unwired: 3 in, 5 out]
            n187 = Bundle By Name(cluster=w387, "VariablePath"=w388, "CreateRefVar.vi"=w382, "DeleteRefVar.vi"=w381) -> (w386:T5)
            n188 = invoke class="VI" method="Save.Instrument"(reference=w392, error in=w391, "Path to saved file"=w381) -> (error out=w389:errorcluster)  [unwired: 3 in, 5 out]
          }
          frame "AddVIsToClass" {
            n189 = Unbundle By Name(w402) -> ("RefVariablesFolderRef"=w411:refnum<vi>, "VariablePath"=w413:path)
            n190 = Unbundle By Name(w402) -> ("CreateRefVar.vi"=w401:path, "DeleteRefVar.vi"=w400:path)
            n191 = invoke class="ProjectItem" method="AddFile"(reference=w411, error in=w412, "Path"=w413) -> (reference out=w408:refnum<vi>, error out=w410:errorcluster)  [unwired: 1 in, 2 out]
            n192 = call <resource>:"CommonVIs_Wait.vi"("error in"=w410) -> ("error out"=w409:errorcluster)  [unwired: 9 in]
            n193 = invoke class="ProjectItem" method="AddFile"(reference=w408, error in=w409, "Path"=w401) -> (error out=w407:errorcluster)  [unwired: 1 in, 3 out]
            n194 = call <resource>:"CommonVIs_Wait.vi"("error in"=w407) -> ("error out"=w406:errorcluster)  [unwired: 9 in]
            n195 = invoke class="ProjectItem" method="AddFile"(reference=w408, error in=w406, "Path"=w400) -> (error out=w405:errorcluster)  [unwired: 1 in, 3 out]
            n196 = call <resource>:"CommonVIs_Wait.vi"("error in"=w405) -> ("error out"=w404:errorcluster)  [unwired: 9 in]
          }
          frame "AddVariableRefToClassPrivateData" {
            n197 = Unbundle By Name(w414) -> ("Data.Name"=w424:string, "Data.DataType"=w422:T1, "Data.Array?"=w426:u16, "VariablePath"=w415:path)  [unwired: 1 out]
            n198 = Concatenate Strings(w424, ".ctl" ("string")) -> (w423:string)
            n199 = call <resource>:"Scripting_PlaceVariableInControl.vi"("ClassRefnum"=w428, "CtlName"=w423, "VariableName"=w424, "DataType"=w422, "ArrayDimension"=w426, "error in"=w430) -> ("error out"=w417:errorcluster)  [unwired: 9 in]
            n200 = Unbundle By Name(w414) -> ("Data.Array?"=w418:u16, "Data.Name"=w420:string, "VariableRef"=w421:refnum<vi>, "Data.DataType"=w419:T1)
            n201 = call <resource>:"Scripting_PlaceDVRRefInObjectAttribute.vi"("Array?"=w418, "ClassRefnum"=w428, "ControlName"=w420, "VariableRef"=w421, "DataType"=w419, "error in"=w417, "AddToObjectAttribute"=FALSE, "TypeDefElement"=w415) -> ("error out"=w429:errorcluster)  [unwired: 11 in]
          }
          frame "UpdateCreateVariableVI" {
            w446 = refnum<vi> refnum  # NamedBundler
            # "Update Class Controls"
            n202 = Unbundle By Name(w443) -> ("CreateRef"=w432:refnum<vi>, "ClassRef"=w458:refnum<vi>, "ClassProvider"=w453:T4)
            n203 = property class="LVClassLibrary"(reference=w458, error in=w456) -> (error out=w454:errorcluster, "Path"=w457:path)  [unwired: 1 out]
            n204 = case shown="\"UnKnown(LabVOOP)\", \"Native\"" w453 {
              tunnel: [_ "object in"] -> w452
              tunnel: [_ "object out"] -> w451
              frame Default {
              }
              frame "UnKnown(LabVOOP)", "Native" {
              }
            }
            n205 = Unbundle By Name(w443) -> ("Data.Name"=w434:string)
            n206 = Path To String(path=w457) -> (string=w455:string)
            n207 = Concatenate Strings(w434, "Ref" ("string")) -> (w433:string)
            n208 = call <resource>:"Scripting_ReplaceOORef.vi"("ViRef"=w432, "NewLvClassFile(ProjectPath or LvClassPath)"=w455, "NewControlLabelName"=w452, "NewIndicatorLabelName"=w451, "error in (no error)"=w454) -> ("error out"=w431:errorcluster)  [unwired: 14 in]
            n209 = Build Array(w433) -> (w442:string[])
            n210 = call <resource>:"Scripting_FindNodeOnDiagram_1.vi"("ViRef(Ignored If Not Wired)"=w432, "NodeTypesToSearchFor"=string[] ["NamedBundler"], "error in (no error)"=w431) -> ("Nodes"=w438:refnum<vi>[], "error out"=w448:errorcluster)  [unwired: 15 in]
            n211 = Bundle(w442) -> (w441:cluster{string[]})  [unwired: 1 in]
            n212 = Index Array(array=w438) -> (element=w447:refnum<vi>)  [unwired: 1 in]
            n213 = Build Array(w441) -> (w440:cluster{string[]}[])
            n214 = To More Specific Class(target class=w446, reference=w447, error in=w448) -> (specific class reference=w445:refnum<vi>, error out=w444:errorcluster)
            n215 = property class="NmdBndl"(reference=w445, error in=w444, "FullElemNms[]"=w440) -> (error out=w439:errorcluster)  [unwired: 1 out]
            n216 = Close Reference(reference=w438, error in (no error)=w439) -> (error out=w437:errorcluster)
            n217 = invoke class="VI" method="Save.Instrument"(reference=w432, error in=w437) -> (error out=w436:errorcluster)  [unwired: 4 in, 5 out]
          }
          frame "UpdateDeleteVariableVI" {
            w477 = refnum<vi> refnum  # NamedUnbundler
            # "Update Class Controls"
            n218 = Unbundle By Name(w474) -> ("DeleteRef"=w462:refnum<vi>, "ClassRef"=w488:refnum<vi>, "ClassProvider"=w483:T4)
            n219 = property class="LVClassLibrary"(reference=w488, error in=w486) -> (error out=w484:errorcluster, "Path"=w487:path)  [unwired: 1 out]
            n220 = case shown="\"UnKnown(LabVOOP)\", \"Native\"" w483 {
              tunnel: [_ "object in"] -> w482
              tunnel: [_ "object out"] -> w481
              frame Default {
              }
              frame "UnKnown(LabVOOP)", "Native" {
              }
            }
            n221 = Path To String(path=w487) -> (string=w485:string)
            n222 = Unbundle By Name(w474) -> ("Data.Name"=w464:string)
            n223 = call <resource>:"Scripting_ReplaceOORef.vi"("ViRef"=w462, "NewLvClassFile(ProjectPath or LvClassPath)"=w485, "NewControlLabelName"=w482, "NewIndicatorLabelName"=w481, "error in (no error)"=w484) -> ("error out"=w461:errorcluster)  [unwired: 14 in]
            n224 = Concatenate Strings(w464, "Ref" ("string")) -> (w463:string)
            n225 = Build Array(w463) -> (w473:string[])
            n226 = call <resource>:"Scripting_FindNodeOnDiagram_1.vi"("ViRef(Ignored If Not Wired)"=w462, "NodeTypesToSearchFor"=string[] ["NamedUnbundler"], "error in (no error)"=w461) -> ("Nodes"=w469:refnum<vi>[], "error out"=w479:errorcluster)  [unwired: 15 in]
            n227 = Bundle(w473) -> (w472:cluster{string[]})  [unwired: 1 in]
            n228 = Index Array(array=w469) -> (element=w478:refnum<vi>)  [unwired: 1 in]
            n229 = Build Array(w472) -> (w471:cluster{string[]}[])
            n230 = To More Specific Class(target class=w477, reference=w478, error in=w479) -> (specific class reference=w476:refnum<vi>, error out=w475:errorcluster)
            n231 = property class="NmdUnbndl"(reference=w476, error in=w475, "FullElemNms[]"=w471) -> (error out=w470:errorcluster)  [unwired: 1 out]
            n232 = Close Reference(reference=w469, error in (no error)=w470) -> (error out=w468:errorcluster)
            n233 = invoke class="VI" method="Save.Instrument"(reference=w462, error in=w468) -> (error out=w467:errorcluster)  [unwired: 4 in, 5 out]
          }
          frame "UpdateIcons" {
            n234 = property class="LVClassLibrary"(reference=w503, error in=w500) -> (reference out=w506:refnum<vi>, error out=w504:errorcluster, "Member Data"=w505:refnum<vi>)
            n235 = Unbundle By Name(w501) -> ("VariableRef"=w502:refnum<vi>, "CreateRef"=w495:refnum<vi>, "DeleteRef"=w491:refnum<vi>)
            n236 = Not A Number/Path/Refnum?(number/path/refnum=w495) -> (NaN/Path/Refnum?=w496:bool)
            n237 = case shown="False" w496 {
              tunnel: w502 -> [w518 w520]
              tunnel: [w517 w519] -> w494
              tunnel: w495 -> [w516 _]
              frame False {
                n238 = Build Array(w518, w516) -> (w517:refnum<vi>[])
              }
              frame True {
                n239 = Build Array(w520) -> (w519:refnum<vi>[])
              }
            }
            n240 = Not A Number/Path/Refnum?(number/path/refnum=w491) -> (NaN/Path/Refnum?=w492:bool)
            n241 = call <resource>:"GDSLvIcon_AnalyseViIcon.vi"("ViRef/LvCLassRef/LvLibRef/ViPath"=w505, "error in (no error)"=w504) -> ("HeaderIcon"=w507:u8[][], "error out"=w498:errorcluster)  [unwired: 5 in, 11 out]
            n242 = case shown="False" w492 {
              tunnel: w494 -> [w514 w515]
              tunnel: [w513 w515] -> w493
              tunnel: w491 -> [w512 _]
              frame False {
                n243 = Build Array (concatenate)(w514, w512) -> (w513:refnum<vi>[])
              }
              frame True {
              }
            }
            n244 = Close Reference(reference=w505, error in (no error)=w498) -> ()  [unwired: 1 out]
            n245 = call <resource>:"GDSLvClass_ReadClassColors.vi"("Library Refnum"=w506, "error in (no error)"=w498) -> ("LvClassIconSettings"=w509:T16, "error out"=w497:errorcluster)  [unwired: 12 in, 4 out]
            n246 = Unbundle By Name(w509) -> ("Frame"=w510:u32, "Frame thickness"=w508:u8)
            n247 = for {
              tunnel: w510 -> [w534]
              tunnel: w508 -> [w533]
              tunnel: w507 -> [w532]
              shift-right: [w525] -> w499
              shift-left: w497 -> [w524]
              tunnel: w493 -> [w521] mode=indexing
              n248 = call <resource>:"GDSLvIcon_AnalyseViIcon.vi"("ViRef/LvCLassRef/LvLibRef/ViPath"=w521, "error in (no error)"=w524) -> ("BodyIcon"=w522:u8[][], "error out"=w523:errorcluster)  [unwired: 5 in, 11 out]
              n249 = call <resource>:"GDSLvIcon_CreateIconPicture.vi"("FrameColor"=w534, "FrameThickness(1)"=w533, "HeaderIconIn"=w532, "BodyIconIn"=w522, "error in (no error)"=w523) -> ("WholeIconOut"=w527:u8[][], "error out"=w530:errorcluster)  [unwired: 9 in, 4 out]
              n250 = Reshape Array(w527, 1024 ("dimension size")) -> (w529:u8[])
              n251 = Bundle By Name(cluster=T11 {"image type"=0, "image depth"=8, "image"=[], "mask"=[], "colors"=[], "Rectangle"={"left"=0, "top"=0, "right"=32, "bottom"=32}} ("image data"), "image"=w529) -> (w531:T11)
              n252 = invoke class="VI" method="VI Icon.Set from Image Data"(reference=w521, error in=w530, "ImageData"=w531) -> (error out=w525:errorcluster)  [unwired: 3 in, 5 out]
            }
          }
          frame "AddCreateVariableVIInCreate" {
            n253 = Unbundle By Name(w536) -> ("Data.AddViToCreate"=w539:bool, "Data.ClassCreateVI"=w538:string)
            n254 = case shown="True" w539 {
              tunnel: w541 -> [w542 w563]
              tunnel: [w542 w562] -> w540
              tunnel: w536 -> [_ w561]
              tunnel: w537 -> [_ w558]
              tunnel: w538 -> [_ w543]
              frame False {
              }
              frame True {
                n255 = Unbundle By Name(w561) -> ("Application"=w556:refnum<vi>, "CreateRef"=w560:refnum<vi>, "ClassProvider"=w559:T4, "TemplateName"=w555:string)
                n256 = property class="LVClassLibrary"(reference=w558) -> ("Path"=w557:path)  [unwired: 1 in, 2 out]
                n257 = To Lower Case(string=w555) -> (all lower case string=w554:string)
                n258 = Strip Path(path=w557) -> (stripped path=w544:path)  [unwired: 1 out]
                n259 = Match Pattern(string=w554, regular expression="singleton") -> (offset past match=w552:i32)  [unwired: 1 in, 3 out]
                n260 = Greater Or Equal To 0?(x=w552) -> (x >= 0?=w551:bool)
                n261 = property class="VI"(reference=w560) -> ("Path"=w548:path)  [unwired: 1 in, 2 out]
                n262 = case shown="\"EndevoGOOP3\", \"EndevoGOOP4\"" w559 {
                  tunnel: ["*Init.vi" w584 "*_Create.vi" "Constructor*.vi"] -> _
                  tunnel: w551 -> [_ w583 _ _]
                  frame "Native", Default {
                  }
                  frame "EndevoGOOP3", "EndevoGOOP4" {
                    n263 = case shown="True" w583 {
                      tunnel: ["*Init.vi" "*_Create.vi"] -> w584
                      frame True {
                      }
                      frame False {
                      }
                    }
                  }
                  frame "OpenG(RootObject)" {
                  }
                  frame "OpenG(OpenG_Object)" {
                  }
                }
                n264 = Build Path(base path=w544, name or relative path=w543) -> (appended path=w545:path)
                n265 = call <vilib>:"Check if File or Folder Exists.vi"("path"=w545) -> ("file or folder exists?"=w546:bool)  [unwired: 8 in, 2 out]
                n266 = Strip Path(path=w548) -> (name=w547:string)  [unwired: 1 out]
                n267 = Format Into String(format string="The \"%s\" could not automatically be placed in the %s method.\nPlease add this method manually." ("message"), w547, w543) -> (resulting string=w549:string)  [unwired: 2 in, 1 out]
                n268 = case shown="True" w546 {
                  tunnel: w563 -> [w564 w566]
                  tunnel: [w564 w567] -> w562
                  tunnel: w548 -> [_ w577]
                  tunnel: w556 -> [_ w575]
                  tunnel: w549 -> [_ w569]
                  tunnel: w545 -> [_ w565]
                  frame False {
                  }
                  frame True {
                    n269 = Open VI Reference(application reference (local)=w575, vi path=w565, error in (no error)=w566) -> (vi reference=w574:refnum<vi>, error out=w576:errorcluster)  [unwired: 3 in]
                    n270 = call <resource>:"Scripting_AddVIInsideNoErrorCase.vi"("ViToModify"=w574, "VIToAdd"=w577, "error in (no error)"=w576, "AddVIOnLeftSideCaseStructure"=FALSE, "OnlyReference"=FALSE) -> ("error out"=w573:errorcluster)  [unwired: 14 in]
                    n271 = invoke class="VI" method="Save.Instrument"(reference=w574, error in=w573) -> (reference out=w571:refnum<vi>, error out=w572:errorcluster)  [unwired: 4 in, 4 out]
                    n272 = Close Reference(reference=w571, error in (no error)=w572) -> (error out=w568:errorcluster)
                    n273 = case shown="Error" w568 {
                      selector: w568 -> [w579 _]
                      tunnel: [w579 w581] -> w567
                      tunnel: w566 -> [_ w581]
                      tunnel: w569 -> [_ w580]
                      frame No Error {
                      }
                      frame Error {
                        n274 = One Button Dialog(message=w580) -> ()  [unwired: 1 in, 1 out]
                      }
                    }
                  }
                }
              }
            }
          }
          frame "AddDeleteVariableVIInDestroy" {
            n275 = Unbundle By Name(w590) -> ("Data.AddViToDelete"=w593:bool, "Data.ClassDestroyVI"=w592:string)
            n276 = case shown="True" w593 {
              tunnel: w595 -> [w596 w617]
              tunnel: [w596 w616] -> w594
              tunnel: w590 -> [_ w615]
              tunnel: w591 -> [_ w613]
              tunnel: w592 -> [_ w597]
              frame False {
              }
              frame True {
                n277 = Unbundle By Name(w615) -> ("Application"=w611:refnum<vi>, "DeleteRef"=w614:refnum<vi>, "ClassProvider"=w602:T4, "TemplateName"=w610:string)
                n278 = property class="LVClassLibrary"(reference=w613) -> ("Path"=w612:path)  [unwired: 1 in, 2 out]
                n279 = To Lower Case(string=w610) -> (all lower case string=w609:string)
                n280 = Strip Path(path=w612) -> (stripped path=w598:path)  [unwired: 1 out]
                n281 = Match Pattern(string=w609, regular expression="singleton") -> (offset past match=w607:i32)  [unwired: 1 in, 3 out]
                n282 = Greater Or Equal To 0?(x=w607) -> (x >= 0?=w599:bool)
                n283 = property class="VI"(reference=w614) -> ("Path"=w604:path)  [unwired: 1 in, 2 out]
                n284 = Build Path(base path=w598, name or relative path=w597) -> (appended path=w601:path)
                n285 = case shown="\"EndevoGOOP3\", \"EndevoGOOP4\"" w602 {
                  tunnel: ["CleanUp.vi" w620 "Destroy.vi" "Destructor*.vi"] -> _
                  tunnel: w599 -> [_ w619 _ _]
                  frame "Native", Default {
                  }
                  frame "EndevoGOOP3", "EndevoGOOP4" {
                    n286 = case shown="False" w619 {
                      tunnel: ["*CleanUp.vi" "Destroy.vi"] -> w620
                      frame True {
                      }
                      frame False {
                      }
                    }
                  }
                  frame "OpenG(RootObject)" {
                  }
                  frame "OpenG(OpenG_Object)" {
                  }
                }
                n287 = call <vilib>:"Check if File or Folder Exists.vi"("path"=w601) -> ("file or folder exists?"=w600:bool)  [unwired: 8 in, 2 out]
                n288 = Strip Path(path=w604) -> (name=w603:string)  [unwired: 1 out]
                n289 = Format Into String(format string="The \"%s\" could not automatically be placed in the %s method.\nPlease add this method manually." ("message"), w603, w597) -> (resulting string=w605:string)  [unwired: 2 in, 1 out]
                n290 = case shown="True" w600 {
                  tunnel: w617 -> [w625 w631]
                  tunnel: [w625 w632] -> w616
                  tunnel: w604 -> [_ w626]
                  tunnel: w611 -> [_ w638]
                  tunnel: w601 -> [_ w637]
                  tunnel: w605 -> [_ w634]
                  tunnel: w599 -> [_ w630]
                  frame False {
                  }
                  frame True {
                    n291 = Open VI Reference(application reference (local)=w638, vi path=w637, error in (no error)=w631) -> (vi reference=w627:refnum<vi>, error out=w629:errorcluster)  [unwired: 3 in]
                    n292 = case shown="True" w630 {
                      tunnel: w626 -> [w643 w650]
                      tunnel: w629 -> [w642 w649]
                      tunnel: w627 -> [w641 w647]
                      tunnel: [w640 w648] -> w628
                      frame False {
                        n293 = call <resource>:"Scripting_AddVIInsideNoErrorCase.vi"("ViToModify"=w641, "VIToAdd"=w643, "error in (no error)"=w642, "AddVIOnLeftSideCaseStructure"=TRUE, "OnlyReference"=TRUE) -> ("error out"=w640:errorcluster)  [unwired: 14 in]
                      }
                      frame True {
                        n294 = call <resource>:"Scripting_AddVIBetweenVIs.vi"("ViToModify"=w647, "VIToAdd"=w650, "VIOne(Path,Name or NamePattern)"="GetInstance.vi" ("regular expression"), "VITwo(Path,Name or NamePattern), If Left/Right-string, it will be placed to the right or left of VIOne"="GetAttributes.vi" ("regular expression"), "error in (no error)"=w649) -> ("error out"=w648:errorcluster)  [unwired: 13 in, 1 out]
                      }
                    }
                    n295 = invoke class="VI" method="Save.Instrument"(reference=w627, error in=w628) -> (reference out=w635:refnum<vi>, error out=w636:errorcluster)  [unwired: 4 in, 4 out]
                    n296 = Close Reference(reference=w635, error in (no error)=w636) -> (error out=w633:errorcluster)
                    n297 = case shown="Error" w633 {
                      selector: w633 -> [w651 _]
                      tunnel: [w651 w653] -> w632
                      tunnel: w631 -> [_ w653]
                      tunnel: w634 -> [_ w652]
                      frame No Error {
                      }
                      frame Error {
                        n298 = One Button Dialog(message=w652) -> ()  [unwired: 1 in, 1 out]
                      }
                    }
                  }
                }
              }
            }
          }
          frame "CloseDown", "CloseRefs", "Error", Default {
            n299 = Unbundle By Name(w663) -> ("DeleteRef"=w660:refnum<vi>, "CreateRef"=w667:refnum<vi>, "VariableRef"=w655:refnum<vi>, "Application"=w664:refnum<vi>, "RefVariablesFolderRef"=w657:refnum<vi>, "Data.Open?"=w656:bool)
            n300 = call <resource>:"GDSError_LogErrorInformation.vi"("State"=w662, "LocalVariableData"=w663, "error in (no error)"=w661) -> ()  [unwired: 16 in, 1 out]
            n301 = case shown="True" w656 {
              tunnel: w655 -> [w669 w672]
              tunnel: [w669 w671] -> w654
              frame False {
              }
              frame True {
                n302 = property class="VI"(reference=w672, "Front Panel.Open"=TRUE ("Front Panel Window:Open")) -> (reference out=w671:refnum<vi>)  [unwired: 1 in, 1 out]
              }
            }
            n303 = stacked-sequence {
              tunnel: w667 -> [w678]
              tunnel: w654 -> [w677]
              tunnel: w664 -> [w676]
              tunnel: w660 -> [w675]
              tunnel: w659 -> [w674]
              tunnel: [w674] -> w658
              tunnel: w657 -> [w673]
              frame #0 {
                n304 = Close Reference(reference=w675) -> ()  [unwired: 1 in, 1 out]
                n305 = Close Reference(reference=w678) -> ()  [unwired: 1 in, 1 out]
                n306 = Close Reference(reference=w677) -> ()  [unwired: 1 in, 1 out]
                n307 = Close Reference(reference=w676) -> ()  [unwired: 1 in, 1 out]
                n308 = Close Reference(reference=w673) -> ()  [unwired: 1 in, 1 out]
              }
            }
            n309 = call <resource>:"GDSLvClass_SaveEverythingInClass.vi"("ClassRefIn"=w658, "ForceResaving(False)"=TRUE, "error in"=w661) -> ("error out"=w665:errorcluster)  [unwired: 15 in, 1 out]
          }
        }
        n310 = Equal?(x=w290, y="Exit") -> (x = y?=w293:bool)
        n311 = Select(t="Error", s=w289, f=w290) -> (s? t:f=w294:string)
      }
    }
    frame "CreatePatternMethod" {
      w684 = "Init"
      n312 = property class="VI"(error in=w681, "Front Panel.Open"=FALSE ("Front Panel Window:Open")) -> (error out=w685:errorcluster)  [unwired: 1 in, 1 out]
      n313 = while {
        shift-right: [w693] -> w680
        shift-left: w685 -> [w700]
        shift-right: [w698] -> _
        shift-left: w684 -> [w699]
        shift-right: [w692] -> _
        shift-left: _ -> [w691]
        tunnel: w683 -> [w690]
        tunnel: w679 -> [w689]
        tunnel: w682 -> [w688]
        shift-left: w684 -> [w687]
        stop <- w697 stop-if-true
        n314 = case shown="\"UpdateBundlers\"" w699 {
          tunnel: w700 -> [w728 w737 w757 w799 w827]
          tunnel: [w720 w735 w765 w790 w827] -> w693
          tunnel: [w719 "ReplaceControlsAndIndicators" "UpdateBundlers" "Exit" "Exit"] -> w694
          tunnel: [w731 w740 w766 w788 w828] -> w692
          tunnel: w691 -> [_ w740 w766 w788 w828]
          tunnel: w690 -> [w730 _ _ _ _]
          tunnel: w689 -> [w729 _ _ _ _]
          tunnel: w688 -> [w721 w738 w756 _ _]
          tunnel: w687 -> [_ _ _ _ _]
          frame "Init" {
            n315 = Variant To Data(error in=w728, type=cluster{path, "VI":refnum<vi>, "Name":string} {path "", "VI"=refnum, "Name"=""} ("cluster"), Variant=w730) -> (data=w711:cluster{path, "VI":refnum<vi>, "Name":string}, error out=w712:errorcluster)
            n316 = Unbundle(w711) -> (w709:path, "VI"=w710:refnum<vi>, "Name"=w701:string)
            n317 = call <resource>:"GDSLvClass_ReadClassType.vi"("Class Refnum In"=w721, "error in (no error)"=w712) -> ("ClassSettings"=w727:T12, "error out"=w720:errorcluster)  [unwired: 15 in, 1 out]
            n318 = Unbundle By Name(w727) -> ("ConnectorPanePattern"=w726:string, "ClassTemplateUsed"=w725:string)
            n319 = To Lower Case(string=w725) -> (all lower case string=w723:string)
            n320 = case shown="\"0\", Default" w726 {
              tunnel: ["4x4x4" "6x8x6"] -> w707
              frame "0", Default {
              }
              frame "1", "2" {
              }
            }
            n321 = Match Pattern(string=w723, regular expression="singleton" ("search string")) -> (offset past match=w724:i32)  [unwired: 1 in, 3 out]
            n322 = Greater Or Equal To 0?(x=w724) -> (x >= 0?=w702:bool)
            n323 = Current VI's Path() -> (path=w717:path)
            n324 = Strip Path(path=w717) -> (stripped path=w716:path)  [unwired: 1 out]
            n325 = Format Into String(format string="ClassAttributes_ReadClassAttributes_%s.vi" ("name or relative path"), w707) -> (resulting string=w713:string)  [unwired: 2 in, 1 out]
            n326 = Build Path(base path=w716, name or relative path="ReferencedVariables_SubVIs") -> (appended path=w705:path)
            n327 = Format Into String(format string="ReferencedVariables_ReadReferencedVariable_%s.vi" ("name or relative path"), w707) -> (resulting string=w708:string)  [unwired: 2 in, 1 out]
            n328 = Build Path(base path=w705, name or relative path=w713) -> ()  [unwired: 1 out]
            n329 = Build Path(base path=w705, name or relative path=w708) -> ()  [unwired: 1 out]
            n330 = Select(t="Find_GetInstanceVI", s=w702, f="ReplaceControlsAndIndicators") -> (s? t:f=w719:string)
            n331 = Bundle By Name(cluster=w729, "MethodTemplate"=w709, "VI"=w710, "Name"=w701, "SupportFolder"=w705, "Singleton"=w702) -> (w731:T5)
          }
          frame "Find_GetInstanceVI" {
            n332 = Unbundle By Name(w740) -> ("VI"=w736:refnum<vi>)
            n333 = call <resource>:"GDSLvClass_GetClassMethod.vi"("Class Refnum In"=w738, "VINames"=string[] ["_GetInstance.vi$"] ("VIsToSerachFor/ViName"), "error in (no error)"=w737) -> ("ViPaths"=w747:path[], "error out"=w742:errorcluster)  [unwired: 13 in, 2 out]
            n334 = call <resource>:"Scripting_FindVisOnDiagram.vi"("ViRef"=w736, "VIsToSerachFor/ViName"=string[] ["ClassAttributes_ReadClassAttributes_4x4x4.vi", "ClassAttributes_ReadClassAttributes_6x8x6.vi"] ("appended array"), "error in (no error)"=w742) -> ("VisFound"=w744:refnum<vi>[], "error out"=w743:errorcluster)  [unwired: 15 in]
            n335 = Index Array(array=w747) -> (element=w741:path)  [unwired: 1 in]
            n336 = Index Array(array=w744) -> (element=w745:refnum<vi>)  [unwired: 1 in]
            n337 = invoke class="GObj" method="Replace"(reference=w745, error in=w743, "Path"=w741) -> (error out=w739:errorcluster, "Replace"=w746:refnum<vi>)  [unwired: 3 in, 4 out]
            n338 = Close Reference(reference=w744, error in (no error)=w739) -> ()  [unwired: 1 out]
            n339 = Close Reference(reference=w746, error in (no error)=w739) -> (error out=w735:errorcluster)
          }
          frame "ReplaceControlsAndIndicators" {
            n340 = Unbundle By Name(w766) -> ("VI"=w762:refnum<vi>, "Name"=w753:string)
            n341 = property class="LVClassLibrary"(reference=w756, error in=w757) -> (error out=w750:errorcluster, "Path"=w759:path)  [unwired: 1 out]
            n342 = property class="VI"(reference=w762) -> ("Panel"=w763:refnum<vi>)  [unwired: 1 in, 2 out]
            n343 = Concatenate Strings(w753, ".ctl" ("string")) -> (w751:string)
            n344 = property class="Pnl"(reference=w763) -> ("Controls[]"=w761:refnum<vi>[])  [unwired: 1 in, 2 out]
            n345 = Strip Path(path=w759) -> (stripped path=w760:path)  [unwired: 1 out]
            n346 = Build Path(base path=w760, name or relative path="ReferencedVariables") -> (appended path=w754:path)
            n347 = Build Path(base path=w754, name or relative path=w751) -> (appended path=w755:path)
            n348 = for {
              tunnel: w761 -> [w773] mode=indexing
              tunnel: w755 -> [w770]
              shift-right: [w774] -> w764
              shift-left: w750 -> [w768]
              n349 = property class="Ctl"(reference=w773, error in=w768) -> (reference out=w771:refnum<vi>, error out=w769:errorcluster, "Label.Text"=w772:string)
              n350 = case shown="\"ReplaceWithtypeDef\"" w772 {
                tunnel: [w775 w779] -> w774
                tunnel: w771 -> [_ w778]
                tunnel: w770 -> [_ w777]
                tunnel: w769 -> [w775 _]
                frame Default {
                }
                frame "ReplaceWithtypeDef" {
                  n351 = invoke class="Ctl" method="Replace"(reference=w778, "Path"=w777) -> (reference out=w776:refnum<vi>, error out=w781:errorcluster, "Replace"=w780:refnum<vi>)  [unwired: 4 in, 3 out]
                  n352 = Close Reference(reference=w780, error in (no error)=w781) -> (error out=w779:errorcluster)
                  n353 = Close Reference(reference=w776, error in (no error)=w781) -> ()  [unwired: 1 out]
                }
              }
            }
            n354 = invoke class="VI" method="Save.Instrument"(reference=w762, error in=w764) -> (error out=w765:errorcluster)  [unwired: 4 in, 5 out]
          }
          frame "UpdateBundlers" {
            n355 = Unbundle By Name(w788) -> ("Name"=w783:string, "VI"=w791:refnum<vi>)
            n356 = call <resource>:"Scripting_FindNodeOnDiagram_1.vi"("ViRef(Ignored If Not Wired)"=w791, "NodeTypesToSearchFor"=string[] ["NamedBundler"], "error in (no error)"=w799) -> ("Nodes"=w798:refnum<vi>[], "error out"=w800:errorcluster)  [unwired: 15 in]
            n357 = Concatenate Strings(w783, "Ref" ("string")) -> (w784:string)
            n358 = Build Array(w784) -> (w787:string[])
            n359 = Bundle(w787) -> (w786:cluster{string[]})  [unwired: 1 in]
            n360 = Build Array(w786) -> (w782:cluster{string[]}[])
            n361 = for {
              tunnel: w798 -> [w822] mode=indexing
              shift-right: [w821] -> w793
              shift-left: w800 -> [w826]
              tunnel: w798 -> [w820] mode=indexing
              tunnel: [w818] -> _
              tunnel: [w817] -> _
              tunnel: w782 -> [w816]
              w825 = refnum<vi> refnum  # NamedBundler
              n362 = To More Specific Class(target class=w825, reference=w820, error in=w826) -> (specific class reference=w824:refnum<vi>, error out=w823:errorcluster)
              n363 = property class="NmdBndl"(reference=w824, error in=w823) -> (reference out=w819:refnum<vi>, error out=w815:errorcluster, "ElemNms[]"=w817:string[], "AvailElems[]"=w818:string[])
              n364 = property class="NmdBndl"(reference=w819, error in=w815, "FullElemNms[]"=w816) -> (error out=w814:errorcluster)  [unwired: 1 out]
              n365 = Close Reference(reference=w822, error in (no error)=w814) -> (error out=w821:errorcluster)
            }
            n366 = call <resource>:"Scripting_FindNodeOnDiagram_1.vi"("ViRef(Ignored If Not Wired)"=w791, "NodeTypesToSearchFor"=string[] ["NamedUnbundler"], "error in (no error)"=w793) -> ("Nodes"=w795:refnum<vi>[], "error out"=w794:errorcluster)  [unwired: 15 in]
            n367 = for {
              tunnel: w795 -> [w810] mode=indexing
              shift-right: [w809] -> w792
              shift-left: w794 -> [w813]
              tunnel: w795 -> [w808] mode=indexing
              tunnel: w782 -> [w805]
              tunnel: [w804] -> _
              tunnel: [w803] -> _
              w807 = refnum<vi> refnum  # NamedUnbundler
              n368 = To More Specific Class(target class=w807, reference=w808, error in=w813) -> (specific class reference=w812:refnum<vi>, error out=w811:errorcluster)
              n369 = property class="NmdUnbndl"(reference=w812, error in=w811) -> (reference out=w806:refnum<vi>, error out=w802:errorcluster, "ElemNms[]"=w803:string[], "AvailElems[]"=w804:string[])
              n370 = property class="NmdUnbndl"(reference=w806, error in=w802, "FullElemNms[]"=w805) -> (error out=w801:errorcluster)  [unwired: 1 out]
              n371 = Close Reference(reference=w810, error in (no error)=w801) -> (error out=w809:errorcluster)
            }
            n372 = invoke class="VI" method="Save.Instrument"(reference=w791, error in=w792) -> (error out=w790:errorcluster)  [unwired: 4 in, 5 out]
          }
          frame Default {
          }
        }
        n373 = Equal?(x=w694, y="Exit") -> (x = y?=w697:bool)
        n374 = Select(t="Error", s=w693, f=w694) -> (s? t:f=w698:string)
      }
    }
    frame "UpdatePattern" {
    }
    frame "RemovePattern" {
    }
  }
  "error out" <- w9
  "DataOut" <- w6
  "Cancelled" <- w7
  "Name" <- w1
  n375 = disable-structure shown="Disabled" {
    frame Disabled {
      (unwired) "CreateDVR1:OpenAndSaveCreateDVR-VI"
      n376 = Select(f="CreateDVR2:AddCreteDVRRefinVI") -> ()  [unwired: 2 in, 1 out]
      n377 = call <resource>:"Scripting_OpenViRef.vi"() -> ()  [unwired: 9 in, 3 out]
    }
    frame Enabled {
    }
  }
